vi "niRFUtil MASMT Resample (constant to constant) (single-channel, CSG).vi"(5 "anti-aliasing?":bool=TRUE, 6 "FIR filter specifications":T1={"alias rejection (dB)"=120.0, "normalized bandwidth"=0.4536}, 7 "reset?":bool, 8 "error in (no error)":errorcluster, 9 "dt":sgl=1.0, 10 "delay":sgl, 11 "X":csg[](array[numeric])) -> (0 "error out":errorcluster, 2 "t0":sgl, 3 "Y":csg[](array[numeric]) format="%#.6g")   [LabVIEW 2015, in "niRFUtil.lvlib"]
doc: "Resamples input signal <B>X</B> according to <B>delay</B> and <B>dt</B> using an FIR filter implementation."
uses:
  niRFUtil.lvlib
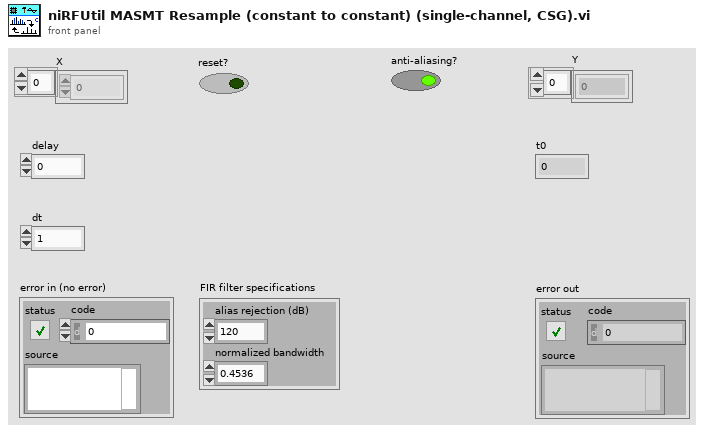
[diagram p1: front panel]
types:
  T1 = cluster{"alias rejection (dB)":sgl, "normalized bandwidth":sgl}
  T2 = cluster{"new sample period":sgl, "first point location":sgl, "timing jitter":i32}
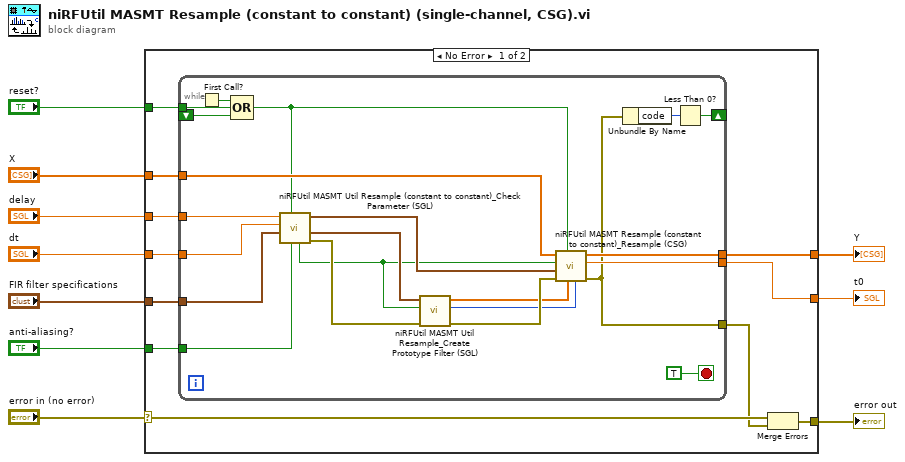
[diagram p0: block diagram]
diagram:
  n1 = case shown="No Error" "error in (no error)" {
    selector: "error in (no error)" -> [w13 w44]
    tunnel: "FIR filter specifications" -> [w14 _]
    tunnel: "dt" -> [w15 _]
    tunnel: "delay" -> [w17 _]
    tunnel: "reset?" -> [w16 _]
    tunnel: "X" -> [w21 _]
    tunnel: "anti-aliasing?" -> [w20 _]
    tunnel: [w11 w44] -> w1
    tunnel: [w19 _] -> w2
    tunnel: [w18 _] -> w3
    frame No Error {
      n2 = while {
        tunnel: w17 -> [w29]
        tunnel: w16 -> [w33]
        tunnel: [w43] -> w19
        tunnel: [w42] -> w18
        tunnel: w15 -> [w28]
        tunnel: w21 -> [w41]
        tunnel: w20 -> [w24]
        tunnel: [w36] -> w12
        shift-right: [w34] -> _
        shift-left: _ -> [w31]
        tunnel: w14 -> [w30]
        stop <- TRUE stop-if-true
        n3 = First Call?() -> (First Call?: T/F=w32:bool)
        n4 = Compound Arithmetic op=OR(w32, w33, w31) -> (w25:bool)
        n5 = call "niRFUtil MASMT Util Resample (constant to constant)_Check Parameter (SGL).vi"("anti-aliasing in"=w24, "reset?"=w25, "FIR filter specifications in"=w30, "dt"=w28, "delay"=w29) -> ("error out"=w26:errorcluster, "FIR filter specifications out"=w23:T1, "config"=w27:T2, "anti-aliasing out"=w22:bool)  [unwired: 3 in]
        n6 = call "niRFUtil MASMT Util Resample_Create Prototype Filter (SGL).vi"("error in (no error)"=w26, "anti-aliasing?"=w22, "FIR filter specifications"=w23) -> ("error out"=w40:errorcluster, "decimation factor"=w38:i32, "Coefficients"=w39:sgl[])  [unwired: 6 in]
        n7 = call "niRFUtil MASMT Resample (constant to constant)_Resample (CSG).vi"("max decimation"=w38, "Resample FIR"=w39, "reset?"=w25, "error in (no error)"=w40, "config"=w27, "anti-aliasing?"=w22, "X"=w41) -> ("error out"=w36:errorcluster, "t0"=w43:sgl, "Y"=w42:csg[])  [unwired: 2 in]
        n8 = Unbundle By Name(w36) -> ("code"=w35:i32)
        n9 = Less Than 0?(x=w35) -> (x < 0?=w34:bool)
      }
      n10 = Merge Errors(w13, w12) -> (w11:errorcluster)
    }
    frame Error {
    }
  }
  "error out" <- w1
  "Y" <- w3
  "t0" <- w2
